vi "Disable Controls.vi"(8 "error in":errorcluster, 11 "refnums in":refnum<vi>[](array[refnum])) -> (0 "error out":errorcluster, 3 "refnums out":refnum<vi>[](array[refnum]))   [LabVIEW 2017]
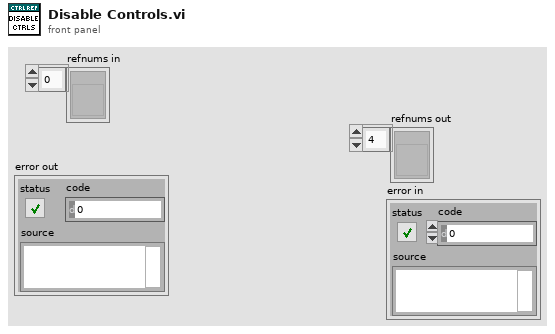
[diagram p1: front panel]
types:
  T1 = enum8{"Enabled", "Disabled", "Disabled and Grayed Out"}
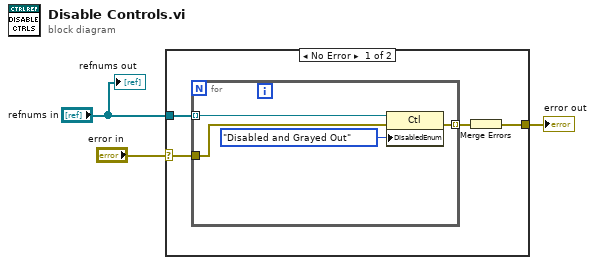
[diagram p0: block diagram]
diagram:
  n1 = case shown="No Error" "error in" {
    selector: "error in" -> [w4 w12]
    tunnel: "refnums in" -> [w6 _]
    tunnel: [w5 w12] -> w2
    frame No Error {
      n2 = for {
        tunnel: w6 -> [w11] mode=indexing
        tunnel: [w9] -> w7 mode=indexing
        tunnel: w4 -> [w10]
        n3 = property class="Ctl"(reference=w11, error in=w10, "DisabledEnum"=T1."Disabled and Grayed Out" ("Disabled")) -> (error out=w9:errorcluster)  [unwired: 1 out]
      }
      n4 = Merge Errors(w7) -> (w5:errorcluster)
    }
    frame Error {
    }
  }
  "error out" <- w2
  "refnums out" <- "refnums in"
